vi "PCO_AddBufferEx.vi"(4 "BitPerPixel":u16=14, 6 "Resolution":cluster{"XRes":u16, "YRes":u16}={"XRes"=1368, "YRes"=1040}, 8 "error in (no error)":errorcluster, 9 "Range":cluster{"1stImage":u32, "LastImage":u32}, 10 "sBufNr":i16, 11 "Handle":u64) -> (0 "error out":errorcluster, 3 "Handle Out":u64, 5 "return type":u32 format="%x")   [LabVIEW 2011]
uses:
  SC2_Cam64.dll
panel:
  # "The input data should be filled with the following parameter:\n• dw1stImage = set to 0 for live view mode(“live view” transfers the most recent image to the \nPC for viewing / monitoring)\n- 0 = live view mode. x = set to the same value as dwLastImage. Has to be a valid image \nnumber (see PCO_GetNumberOfImagesInSegment, 1…max available).\n• dwLastImage = set to 0 in preview mode.\n- 0 = live view mode. x = set to the same value as dw1stImage. Has to be a valid image \nnumber (see PCO_GetNumberOfImagesInSegment, 1…max available).\n• sBufNr: 0 … 7:.number of desired buffer. A buffer can be reused after the event is fired.\n• wXRes: Actual x-Resolution of the image which should be transferred.\n• wYRes: Actual y-Resolution of the image which should be transferred.\n• WBitPerPixel: BitResolution of the image which should be transferred."
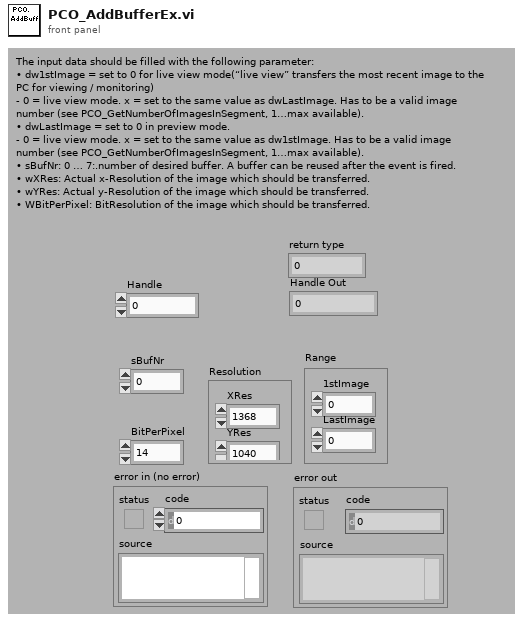
[diagram p1: front panel]
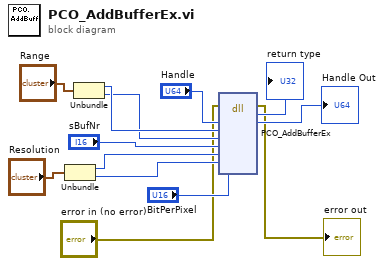
[diagram p0: block diagram]
diagram:
  n1 = Unbundle("Resolution") -> ("XRes"=w4:u16, "YRes"=w3:u16)
  n2 = Unbundle("Range") -> ("1stImage"=w7:u32, "LastImage"=w6:u32)
  n3 = dll-call lib="C:/Program Files/colibri/Drivers/PCO.Camera/SC2_Cam*.*" fn="PCO_AddBufferEx"(error in="error in (no error)", "Handle"="Handle", "1stImage"=w7, "LastImage"=w6, "sBufNr"="sBufNr", "XRes"=w4, "YRes"=w3, "BitPerPixel"="BitPerPixel") -> (error out=→"error out":errorcluster, "return type"=→"return type":u32, "Handle"=→"Handle Out":u64)  [unwired: 8 in, 1 out]
